vi "Destroy.vi"(8 "error in (no error)":errorcluster, 11 "Object In":refnum<class "Object.lvclass">) -> (0 "error out":errorcluster, 3 "Object Out":refnum<class "Object.lvclass">)   [LabVIEW 2015, in "Front Panel Publisher.lvlib" / "Object.lvclass"]
uses:
  Object.lvclass
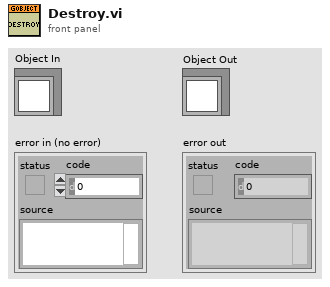
[diagram p1: front panel]
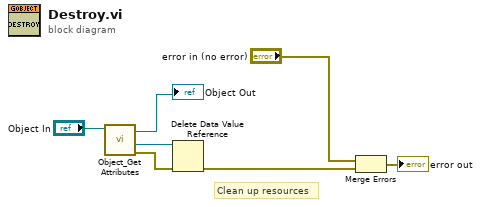
[diagram p0: block diagram]
diagram:
  # "Clean up resources"
  n1 = call "Object_Get Attributes.vi"("Object In"="Object In") -> ("error out"=w4:errorcluster, "DataRef"=w3:refnum<data-value>, "Object Out"=→"Object Out":refnum<class "Object.lvclass">)  [unwired: 7 in, 1 out]
  n2 = Delete Data Value Reference(data value reference=w3, error in=w4) -> (error out=w1:errorcluster)  [unwired: 1 out]
  n3 = Merge Errors("error in (no error)", w1) -> (→"error out":errorcluster)
